vi "GFITS_GetStatFmList.vi"(9 "List In":string[][](table), 10 "status":string) -> (1 "List Out":string[][](table))   [LabVIEW 2016]
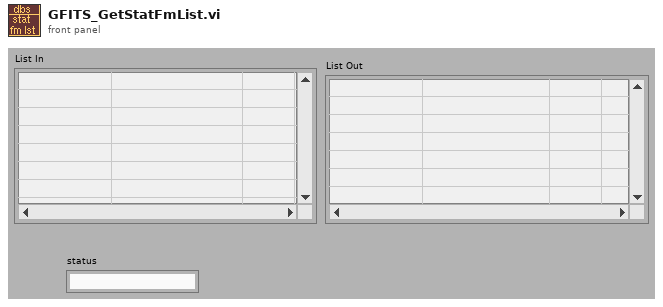
[diagram p1: front panel]
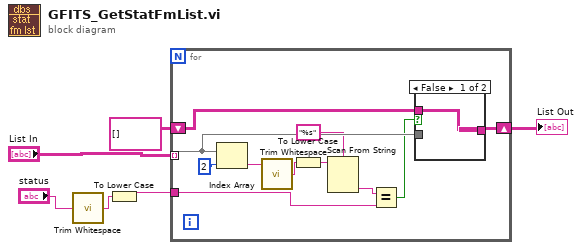
[diagram p0: block diagram]
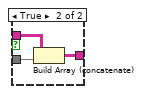
[diagram p2: hidden frame]
diagram:
  n1 = call <vilib>:"Trim Whitespace.vi"("string"="status") -> ("trimmed string"=w3:string)  [unwired: 1 in]
  n2 = To Lower Case(string=w3) -> (all lower case string=w1:string)
  n3 = for {
    tunnel: "List In" -> [w16] mode=indexing
    shift-right: [w15] -> w2
    shift-left: string[][] [] -> [w14]
    tunnel: w1 -> [w10]
    n4 = Index Array(array=w16, index=2) -> (element=w13:string)
    n5 = call <vilib>:"Trim Whitespace.vi"("string"=w13) -> ("trimmed string"=w12:string)  [unwired: 1 in]
    n6 = To Lower Case(string=w12) -> (all lower case string=w9:string)
    n7 = Scan From String(format string="%s", input string=w9) -> (output 1=w7:string)  [unwired: 2 in, 4 out]
    n8 = Equal?(x=w7, y=w10) -> (x = y?=w11:bool)
    n9 = case shown="False" w11 {
      tunnel: w16 -> [_ w21]
      tunnel: [w18 w20] -> w15
      tunnel: w14 -> [w18 w19]
      frame False {
      }
      frame True {
        n10 = Build Array (concatenate)(w19, w21) -> (w20:string[][])
      }
    }
  }
  "List Out" <- w2
